vi "触发拍照CCD2.vi"(8 "error in":errorcluster, 9 "曝光值":i64=500 caption="ValueI64" min=500 max=5000000, 10 "Image Name":string="untitled", 11 "Session In":T2) -> (0 "error out":errorcluster, 1 "Buffer Number Out":u32, 2 "Image Out 3":T1(plugin-control), 3 "Session Out":T2)   [LabVIEW 2017]
uses:
  <vilib>/userdefined/High Color/IMAQdx.ctl
  <vilib>/vision/driver/NI_Vision_Acquisition_Software.lvlib
  <resource>/objmgr/imaqdx.rc
  <vilib>/vision/driver/IMAQdx.llb/IMAQdx Camera Control Mode.ctl
panel:
  out "error out 2":errorcluster caption="错误输出"
  in  "error in (no error)":errorcluster caption="错误输入（无错误）"
  out "TrgCnt out 2":i32
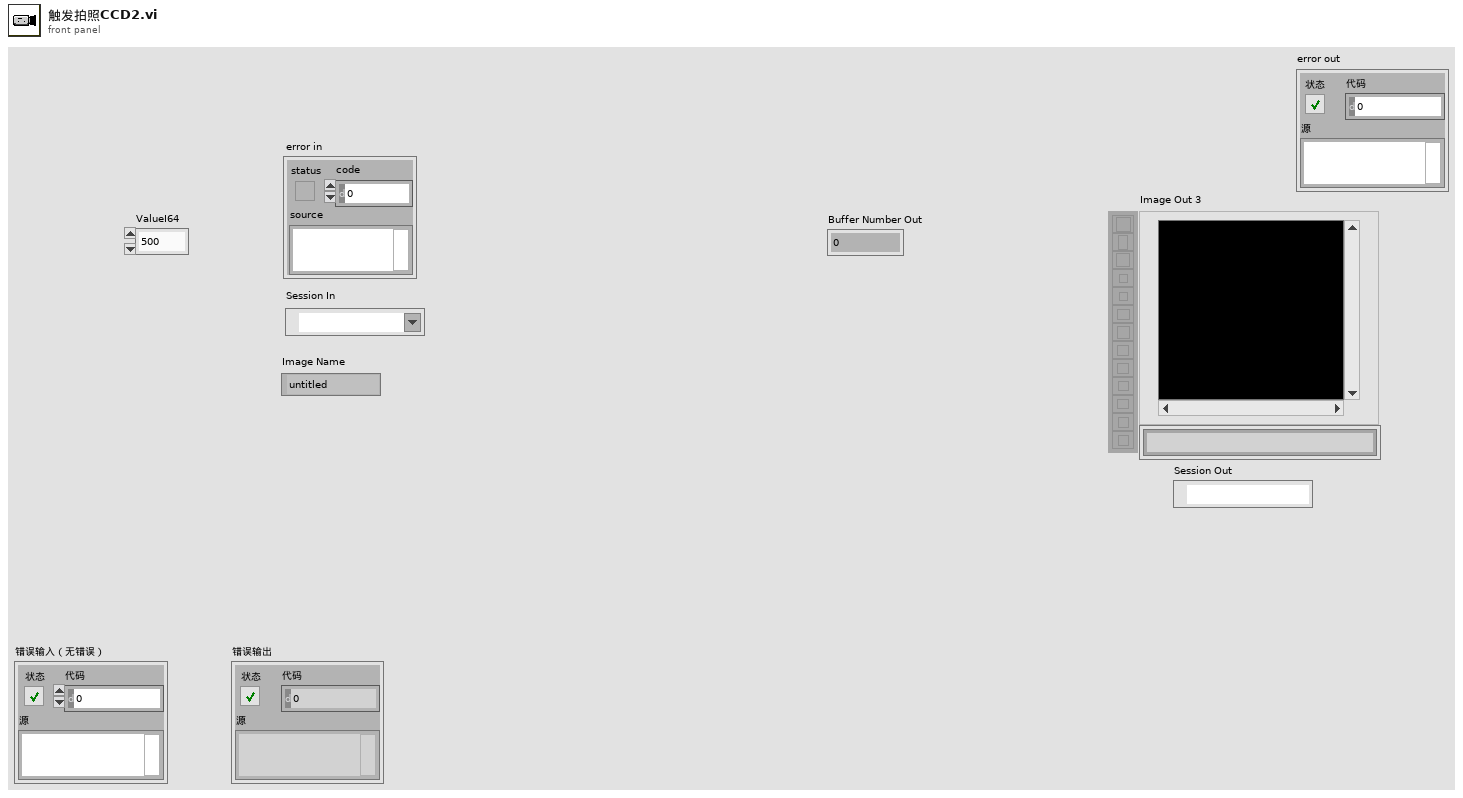
[diagram p1: front panel]
types:
  T1 = typedef "IMAQ Image.ctl" = refnum<image>
  T2 = typedef "IMAQdx.ctl" = refnum<k21>
  T3 = typedef "Image Type" = u32
  T4 = typedef "NI_Vision_Acquisition_Software.lvlib/IMAQdx Camera Control Mode.ctl" = enum32{"Controller", "Listener"}
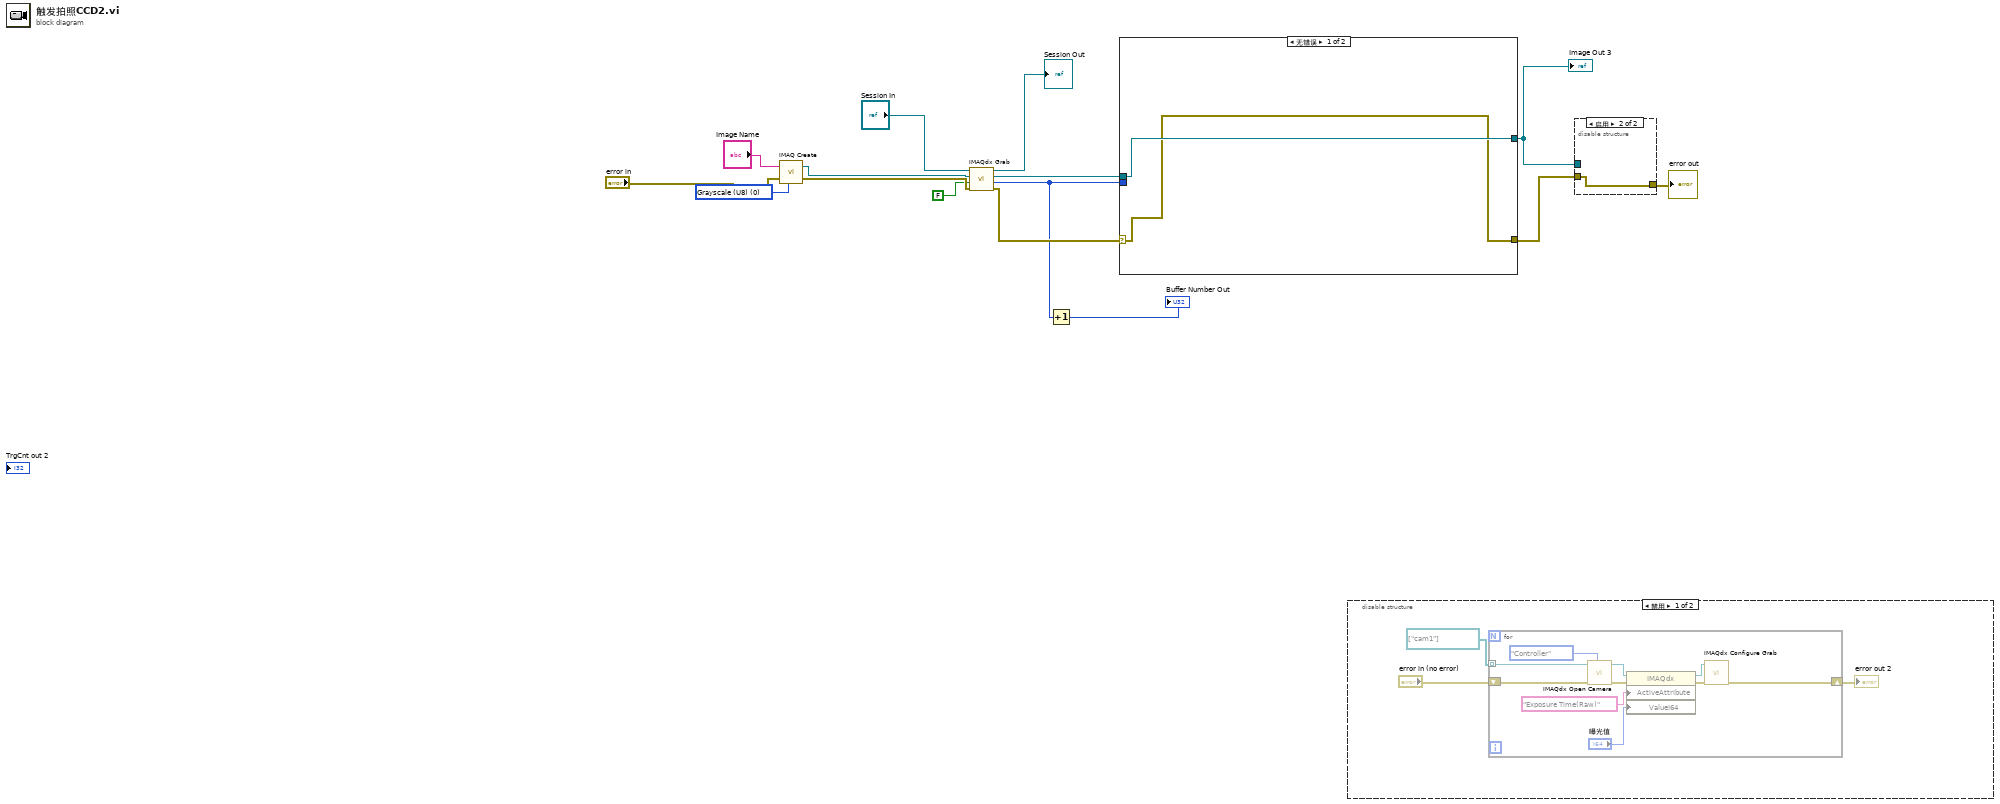
[diagram p0: block diagram]
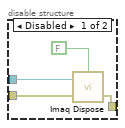
[diagram p3: hidden frame]
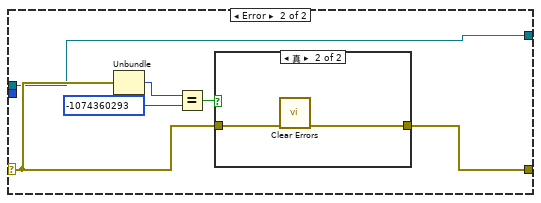
[diagram p4: hidden frame]
diagram:
  w6 = T3 0 items=["Grayscale (U8)", "Grayscale (I16)", "Grayscale (SGL)", "Complex (CSG)", "RGB (U32)", "HSL (U32)", "RGB (U64)", "Grayscale (U16)"] ("Image Type")
  n1 = call "IMAQ Create"("Image Name"="Image Name", "Image Type"=w6, "error in (no error)"="error in") -> ("New Image"=w9:T1, "error out"=w10:errorcluster)  [unwired: 2 in]
  n2 = call <vilib>:"IMAQdx Grab.vi"("error in"=w10, "Wait for Next Buffer? (Yes)"=FALSE, "Image In"=w9, "Session In"="Session In") -> ("error out"=w14:errorcluster, "Buffer Number Out"=w7:u32, "Image Out"=w8:T1, "Session Out"=→"Session Out":T2)  [unwired: 4 in]
  n3 = Increment(x=w7) -> (x+1=→"Buffer Number Out":u32)
  n4 = case shown="无错误" w14 {
    selector: w14 -> [w16 w23]
    tunnel: [w16 w22] -> w4
    tunnel: w8 -> [w17 w18]
    tunnel: [w17 w18] -> w2
    tunnel: w7 -> [_ _]
    frame No Error {
    }
    frame Error {
      n5 = Unbundle(w23) -> ("code"=w21:i32)  [unwired: 2 out]
      n6 = Equal?(x=w21, y=-1074360293) -> (x = y?=w20:bool)
      n7 = case shown="真" w20 {
        tunnel: w23 -> [w24 w26]
        tunnel: [w24 w25] -> w22
        frame False {
        }
        frame True {
          n8 = call <vilib>:"Clear Errors.vi"("error in (no error)"=w26) -> ("error out"=w25:errorcluster)  [unwired: 5 in, 1 out]
        }
      }
    }
  }
  "Image Out 3" <- w2
  n9 = disable-structure shown="禁用" {
    frame Disabled {
      n10 = for {
        tunnel: T2[] ["cam1"] -> [w30] mode=indexing
        shift-right: [w32] -> w29
        shift-left: "error in (no error)" -> [w31]
        n11 = call <vilib>:"IMAQdx Open Camera.vi"("Camera Control Mode"=IMAQdx_Camera_Control_Mode."Controller", "error in"=w31, "Session In"=w30) -> ("error out"=w36:errorcluster, "Session Out"=w37:T2)  [unwired: 7 in]
        n12 = property class="IMAQdx"(reference=w37, error in=w36, "ActiveAttribute"="Exposure Time(Raw)", "ValueI64"="曝光值") -> (reference out=w34:T2, error out=w33:errorcluster)
        n13 = call <vilib>:"IMAQdx Configure Grab.vi"("error in"=w33, "Session In"=w34) -> ("error out"=w32:errorcluster)  [unwired: 8 in, 1 out]
      }
      "error out 2" <- w29
    }
    frame Enabled {
    }
  }
  n14 = disable-structure shown="启用" {
    disable-tunnel: w4 -> [w43 w44]
    disable-tunnel: [w42 w44] -> w3
    disable-tunnel: w2 -> [w40 _]
    frame Disabled {
      n15 = call "Imaq Dispose"("All Images? (No)"=FALSE, "Image"=w40, "error in (no error)"=w43) -> ("error out"=w42:errorcluster)  [unwired: 3 in]
    }
    frame Enabled {
    }
  }
  "error out" <- w3
